vi "Final_project_baseline.vi"() -> ()   [LabVIEW 2019]
uses:
  <vilib>/sound2/lvsound2.llb/Sampling Mode.ctl
  <vilib>/sound2/lvsound2.llb/Sound Data Format.ctl
  <vilib>/imath/engines/lvmath2/RunTimeEngine/Managers/WorkSpace/UID Generator.vi
  <vilib>/imath/engines/lvmath2/RunTimeEngine/BuiltInFunctions/sum/NIMS_sum(GV).vi
  <instcachedir>/0/NIMS_sum(GV)_67F5EC36BC034E54A6BEC5B0673C00E5.lvgen/NIMS_sum(GV)_67F5EC36BC034E54A6BEC5B0673C00E5_000.vi
  <vilib>/imath/engines/lvmath2/RunTimeEngine/RunTimeType/NIMS_RunTimeType_From StrictType (excl LVString).vi
  <instcachedir>/0/NIMS_RunTimeType_From StrictType (excl LVString)_D8AFBA86A94845AAA577C895450664BD.lvgen/NIMS_RunTimeType_From StrictType (excl LVString)_D8AFBA86A94845AAA577C895450664BD_000.vi
  <vilib>/imath/engines/lvmath2/RunTimeEngine/LocalVariableDefStatement/MC_LocalVariableDefStatement_Display.vi
  <vilib>/imath/engines/lvmath2/RunTimeSupport/NIMS_Error if Not Equal.vi
  <instcachedir>/0/NIMS_Error if Not Equal_D50A0F08CBFC40E0B64682CCD852CBC7.lvgen/NIMS_Error if Not Equal_D50A0F08CBFC40E0B64682CCD852CBC7_000.vi
  <vilib>/imath/engines/lvmath2/RunTimeEngine/IndexRead/NIMS V(S).vi
  <instcachedir>/0/NIMS V(S)_0488751826AF41519A22953C041130DC.lvgen/NIMS V(S)_0488751826AF41519A22953C041130DC_000.vi
  <vilib>/imath/engines/lvmath2/RunTimeEngine/ErrorHandling/NIMS_Create Error From Enums.vi
  <vilib>/imath/engines/lvmath2/RunTimeEngine/Managers/SymbolTable/Clear UID.vi
  <vilib>/imath/engines/lvmath2/RunTimeEngine/NodeEndStatement/NIMS_NodeEndStatement_Output.vi
  <instcachedir>/0/NIMS_NodeEndStatement_Output_53EC0D466D134D7ABD903AC30B43404B.lvgen/NIMS_NodeEndStatement_Output_53EC0D466D134D7ABD903AC30B43404B_001.vi
  <vilib>/imath/engines/lvmath2/RunTimeEngine/ErrorHandling/NIMS_Finalize Error.vi
  <vilib>/sound2/lvsound2.llb/Sound Output Write (DBL).vi
  <vilib>/imath/engines/lvmath2/RunTimeEngine/Managers/SymbolTable/NIMS_WorkSpace.lvlib
panel:
  out "Note Index":dbl
  out "Note Frequency":dbl
  in  "Song Notes":dbl[](array[numeric])
  out "Note Wavelength":dynamicdata(graph)
  in  "Amplitude":dbl(slide)=1.0 scale=0.0..10.0
  in  "stop":bool
  out "Waveform Chart":dbl[][](graph)
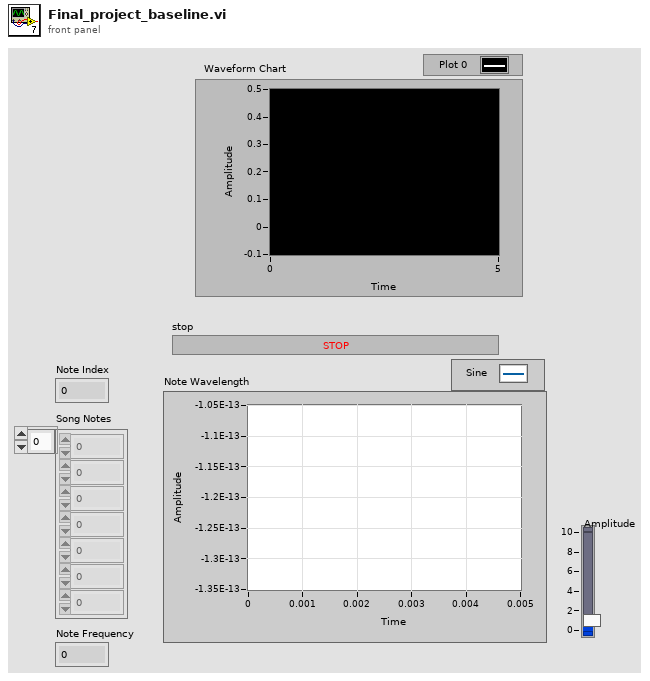
[diagram p1: front panel]
types:
  T1 = typedef "Sound Data Format.ctl" = cluster{"sample rate (S/s)":dbl, "number of channels":i32, "bits per sample":i32}
  T2 = typedef "Sampling Mode.ctl" = i32
  T3 = typedef "Sound Output Task ID.ctl" = u32
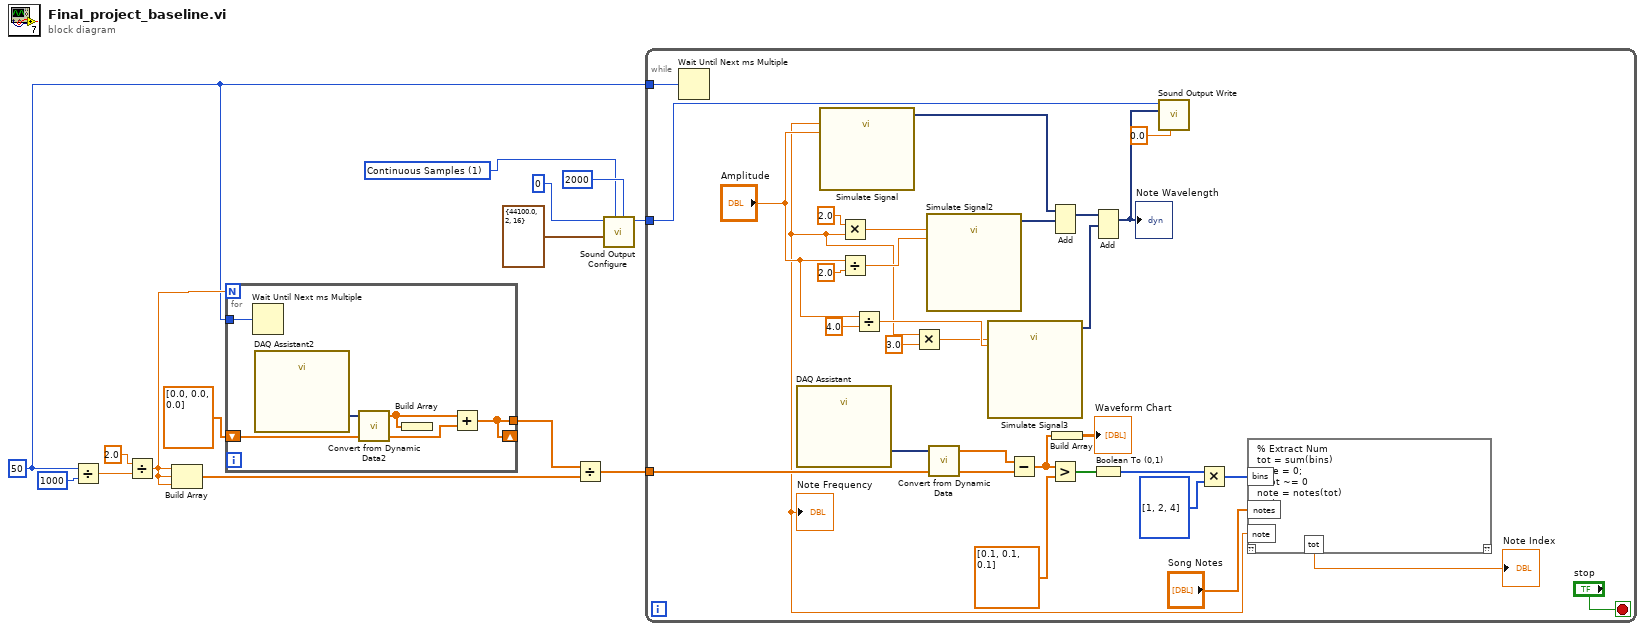
[diagram p0: block diagram]
diagram:
  w1 = u32 50 ("millisecond multiple")
  w13 = T2 1 items=["Finite Samples", "Continuous Samples"] ("sample mode")
  n1 = Divide(x=w1, y=u32 1000) -> (x/y=w8:dbl)
  n2 = Divide(x=2.0, y=w8) -> (x/y=w2:dbl)
  n3 = Build Array(w2, w2, w2) -> (w3:dbl[])
  n4 = for {
    N: w2 -> [_]
    tunnel: w1 -> [w19]
    shift-right: [w16] -> _
    shift-left: dbl[] [0.0, 0.0, 0.0] -> [w18]
    tunnel: [w16] -> w6
    n5 = Wait Until Next ms Multiple(millisecond multiple=w19) -> ()  [unwired: 1 out]
    n6 = call "DAQ Assistant2"() -> ("data"=w17:dynamicdata)  [unwired: 17 in, 2 out]
    n7 = call "Convert from Dynamic Data2"("Dynamic Data Type"=w17) -> ("Array"=w15:dbl[])  [unwired: 3 in]
    n8 = Build Array(w15) -> ()  [unwired: 1 out]
    n9 = Add(x=w15, y=w18) -> (x+y=w16:dbl[])
  }
  n10 = Divide(x=w6, y=w3) -> (x/y=w7:dbl[])
  n11 = call <vilib>:"Sound Output Configure.vi"("number of samples/ch"=2000, "sample mode"=w13, "sound format"=T1 {"sample rate (S/s)"=44100.0, "number of channels"=2, "bits per sample"=16}, "device ID"=u32 0) -> ("task ID"=w10:T3)  [unwired: 6 in, 1 out]
  n12 = while {
    tunnel: w1 -> [w49]
    tunnel: w10 -> [w48]
    tunnel: w7 -> [w35]
    stop <- "stop" stop-if-true
    n13 = Wait Until Next ms Multiple(millisecond multiple=w49) -> ()  [unwired: 1 out]
    n14 = call "DAQ Assistant"() -> ("data"=w29:dynamicdata)  [unwired: 17 in, 2 out]
    n15 = Divide(x="Amplitude", y=2.0) -> (x/y=w44:dbl)
    n16 = Divide(x="Amplitude", y=4.0) -> (x/y=w23:dbl)
    n17 = call "Convert from Dynamic Data"("Dynamic Data Type"=w29) -> ("Array"=w32:dbl[])  [unwired: 3 in]
    n18 = Subtract(x=w32, y=w35) -> (x-y=w34:dbl[])
    n19 = Greater?(x=w34, y=dbl[] [0.1, 0.1, 0.1]) -> (0:w39:bool[])
    n20 = Build Array(w34) -> (→"Waveform Chart":dbl[][])
    n21 = Boolean To (0,1)(Boolean=w39) -> (0, 1=w37:i16[])
    n22 = Multiply(x=w37, y=i32[] [1, 2, 4]) -> (x*y=w36:i32[])
    n23 = mathscript code="% Extract Num\ntot = sum(bins)\nnote = 0;\nif tot ~= 0\nnote = notes(tot)\nend"("bins"=w36, "notes"="Song Notes") -> ("note"=w22:dbl, "tot"=→"Note Index":dbl)  [unwired: 1 in, 1 out]
    "Note Frequency" <- w22
    n24 = call "Simulate Signal"("Frequency"=w22, "Amplitude"="Amplitude") -> ("Sine"=w46:dynamicdata)  [unwired: 12 in, 1 out]
    n25 = Multiply(x=2.0, y=w22) -> (x*y=w43:dbl)
    n26 = Multiply(x=w22, y=3.0) -> (x*y=w20:dbl)
    n27 = call "Simulate Signal2"("Frequency"=w43, "Amplitude"=w44) -> ("Sine"=w47:dynamicdata)  [unwired: 12 in, 1 out]
    n28 = call "Simulate Signal3"("Frequency"=w20, "Amplitude"=w23) -> ("Sine"=w28:dynamicdata)  [unwired: 12 in, 1 out]
    n29 = Add(1:w47, 2:w46) -> (0:w27:dynamicdata)  [unwired: 1 in, 1 out]
    n30 = Add(1:w28, 2:w27) -> (0:w26:dynamicdata)  [unwired: 1 in, 1 out]
    "Note Wavelength" <- w26
    n31 = call-poly <vilib>:"Sound Output Write.vi"("timeout (sec)"=0.0, "data"=w26, "task ID"=w48) -> ()  [unwired: 7 in, 2 out]
  }
